vi "SetUIState.vi"(8 "error in (no error)":errorcluster, 10 "UI State":T1=enum."Embedded", 11 "EmbeddedSMO in":refnum<class "SMO.UI.Embedded.lvclass">) -> (0 "error out":errorcluster, 3 "EmbeddedSMO out":refnum<class "SMO.UI.Embedded.lvclass">)   [LabVIEW 2019, in "SMO.UI.Embedded.lvclass"]
uses:
  SMO.UI.Embedded.lvclass
  Typedefs/UI State.ctl
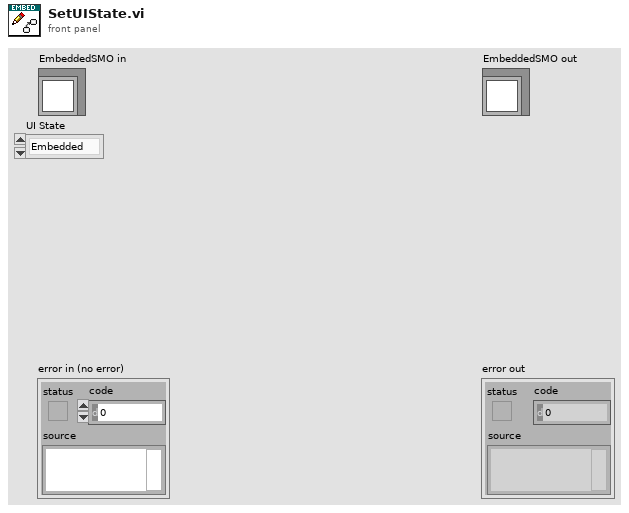
[diagram p1: front panel]
types:
  T1 = typedef "SMO.UI.Embedded.lvclass/UI State.ctl" = enum16{"unknown", "Opened", "Embedded", "Closed"}
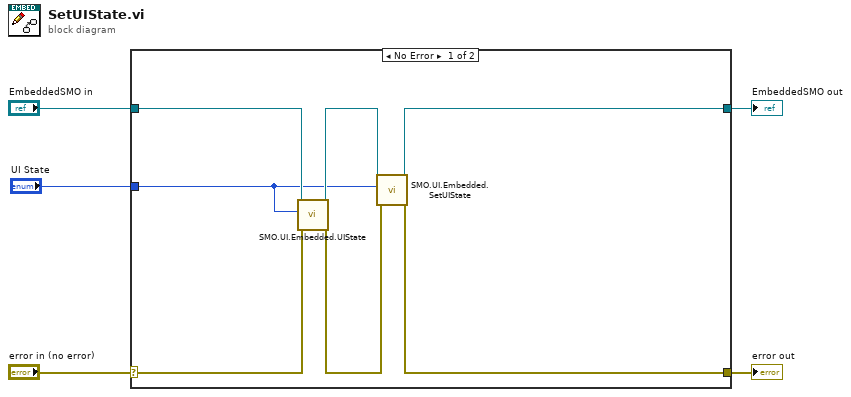
[diagram p0: block diagram]
diagram:
  n1 = case shown="No Error" "error in (no error)" {
    selector: "error in (no error)" -> [w6 w14]
    tunnel: [w11 w14] -> w4
    tunnel: [w12 w13] -> w2
    tunnel: "EmbeddedSMO in" -> [w9 w13]
    tunnel: "UI State" -> [w7 _]
    frame No Error {
      n2 = call "SMO.UI.Embedded.UIState.vi"("error in (no error)"=w6, "UI State"=w7, "SMO.UI.Embedded"=w9) -> ("error out"=w8:errorcluster, "SMO.UI.Embedded out"=w10:refnum<class "SMO.UI.Embedded.lvclass">)  [unwired: 7 in]
      n3 = call "SMO.UI.Embedded.SetUIState.vi"("error in (no error)"=w8, "UI State"=w7, "EmbeddedSMO"=w10) -> ("error out"=w11:errorcluster, "EmbeddedSMO out"=w12:refnum<class "SMO.UI.Embedded.lvclass">)  [unwired: 7 in]
    }
    frame Error {
    }
  }
  "error out" <- w4
  "EmbeddedSMO out" <- w2
